vi "Flipper Control Servo.vi"(3 "Cannon Position(deg)":dbl, 4 "Enable Stack":bool, 5 "override flipper":bool) -> (0 "Stop Conveyer Belt":bool, 1 "Set Flipper's Servos Angle":i32)   [LabVIEW 2012]
uses:
  BotStatus.vi
panel:
  # "Flipper Angle"
  # "Cannon Angle"
  # "90"
  # "90-min / 90"
  # "170"
  # "0 / min angle"
  # "90 / min+90"
  # "48.6 => 49"
  # "-min angle / 0"
  # "0"
  # "original angle / \"Cannon Position(deg)\""
  # "FlipperAtPlace is True if the servo is at 0 degrees"
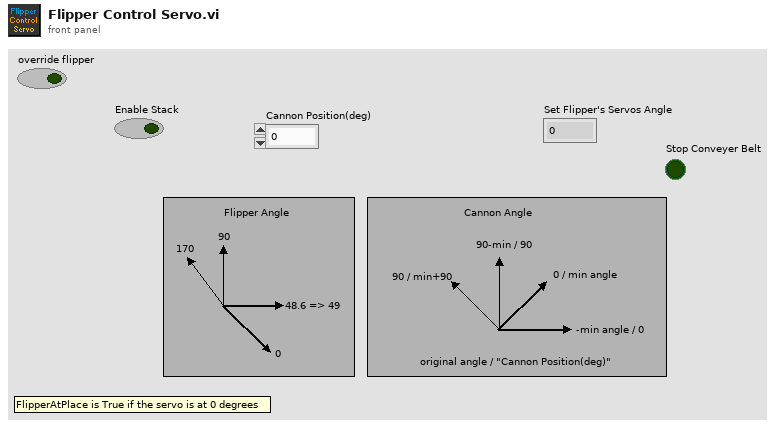
[diagram p1: front panel]
types:
  T1 = cluster{"Middle":bool, "InCannon":bool, "InFlipper":bool, "Bottom":bool, "FlipperDown":bool}
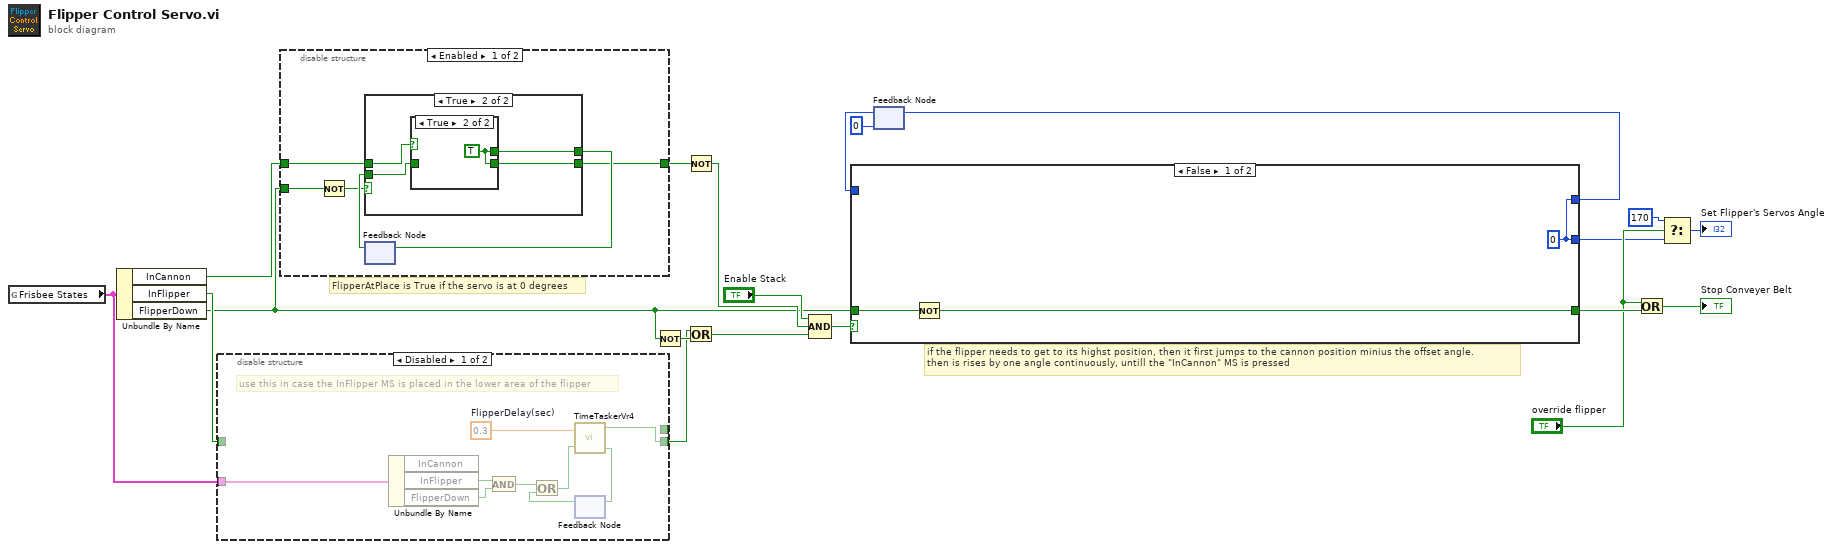
[diagram p0: block diagram]
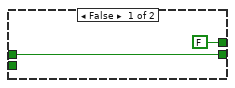
[diagram p3: hidden frame]
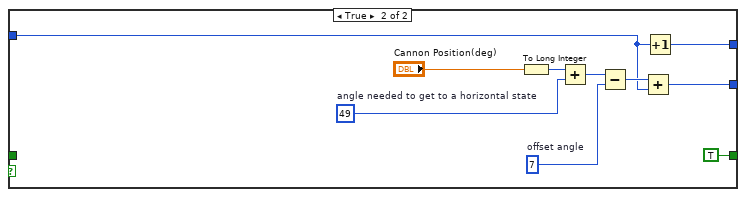
[diagram p6: hidden frame]
diagram:
  # "FlipperAtPlace is True if the servo is at 0 degrees"
  # "if the flipper needs to get to its highst position, then it first jumps to the cannon position minius the offset angle.\nthen is rises by one angle continuously, untill the \"InCannon\" MS is pressed"
  n1 = global read "BotStatus.vi" "Frisbee States"() -> (w1:T1)
  n2 = Unbundle By Name(w1) -> ("InCannon"=w4:bool, "InFlipper"=w3:bool, "FlipperDown"=w2:bool)
  n3 = disable-structure shown="Disabled" {
    disable-tunnel: [w24 w30] -> w11
    disable-tunnel: [_ w30] -> _
    disable-tunnel: w3 -> [_ w30]
    disable-tunnel: w1 -> [w21 _]
    frame Disabled {
      w25 = 0.3  # FlipperDelay(sec)
      # "use this in case the InFlipper MS is placed in the lower area of the flipper"
      n4 = Unbundle By Name(w21) -> ("InFlipper"=w22:bool, "FlipperDown"=w23:bool)  [unwired: 1 out]
      n5 = And(x=w22, y=w23) -> (x .and. y?=w29:bool)
      n6 = feedback #1() -> (w28:bool)  [unwired: 1 in]
      n7 = Or(x=w29, y=w28) -> (x .or. y?=w26:bool)
      n8 = call "TimeTaskerVr4.vi"("Delay(sec)"=w25, "Start Counting?"=w26) -> ("TimePast?"=w24:bool, "Counting?"=w27:bool)  [unwired: 1 out]
      n9 = feedback-in #1(w27) -> ()
    }
    frame Enabled {
    }
  }
  n10 = disable-structure shown="Enabled" {
    disable-tunnel: w2 -> [w33 _]
    disable-tunnel: w4 -> [w32 w45]
    disable-tunnel: [w31 w45] -> w12
    frame Enabled {
      n11 = Not(x=w33) -> (.not. x?=w34:bool)
      n12 = feedback #2() -> (w35:bool)  [unwired: 1 in]
      n13 = case shown="True" w34 {
        tunnel: [w38 w39] -> w31
        tunnel: w32 -> [w38 w42]
        tunnel: [FALSE w41] -> w36
        tunnel: w35 -> [_ w40]
        frame False {
        }
        frame True {
          n14 = case shown="True" w42 {
            tunnel: [w43 w44] -> w41
            tunnel: w40 -> [w43 _]
            tunnel: [w43 w44] -> w39
            frame False {
            }
            frame True {
              w44 = TRUE
            }
          }
        }
      }
      n15 = feedback-in #2(w36) -> ()
    }
    frame Disabled {
      # "use this in case the InCannon MS is\nplaced on the flipper at all time"
    }
  }
  n16 = Not(x=w2) -> (.not. x?=w18:bool)
  n17 = Not(x=w12) -> (.not. x?=w20:bool)
  n18 = Or(x=w11, y=w18) -> (x .or. y?=w19:bool)
  n19 = Compound Arithmetic op=AND("Enable Stack", w20, w19) -> (w10:bool)
  n20 = feedback #3(0) -> (w16:i32)
  n21 = case shown="False" w10 {
    tunnel: [w48 w52] -> w7
    tunnel: [w48 w53] -> w17
    tunnel: w16 -> [_ w51]
    tunnel: [w46 TRUE ("Stop Conveyer Belt")] -> w14
    tunnel: w2 -> [w47 _]
    frame False {
      w48 = 0
      n22 = Not(x=w47) -> (.not. x?=w46:bool)
    }
    frame True {
      w58 = 49  # angle needed to get to a horizontal state
      w56 = 7  # offset angle
      n23 = To Long Integer(number="Cannon Position(deg)") -> (32bit integer=w55:i32)
      n24 = Add(x=w55, y=w58) -> (x+y=w57:i32)
      n25 = Subtract(x=w57, y=w56) -> (x-y=w54:i32)
      n26 = Add(x=w54, y=w51) -> (x+y=w52:i32)
      n27 = Increment(x=w51) -> (x+1=w53:i32)
    }
  }
  n28 = feedback-in #3(w17) -> ()
  n29 = Or(x="override flipper", y=w14) -> (x .or. y?=→"Stop Conveyer Belt":bool)
  n30 = Select(t=170, s="override flipper", f=w7) -> (s? t:f=→"Set Flipper's Servos Angle":i32)
